vi "多反-初始化img句柄.vi"(11 "idx":i32) -> (3 "imgDFs":T2)   [LabVIEW 2018]
uses:
  <vilib>/vision/Image Controls.llb/IMAQ Image.ctl
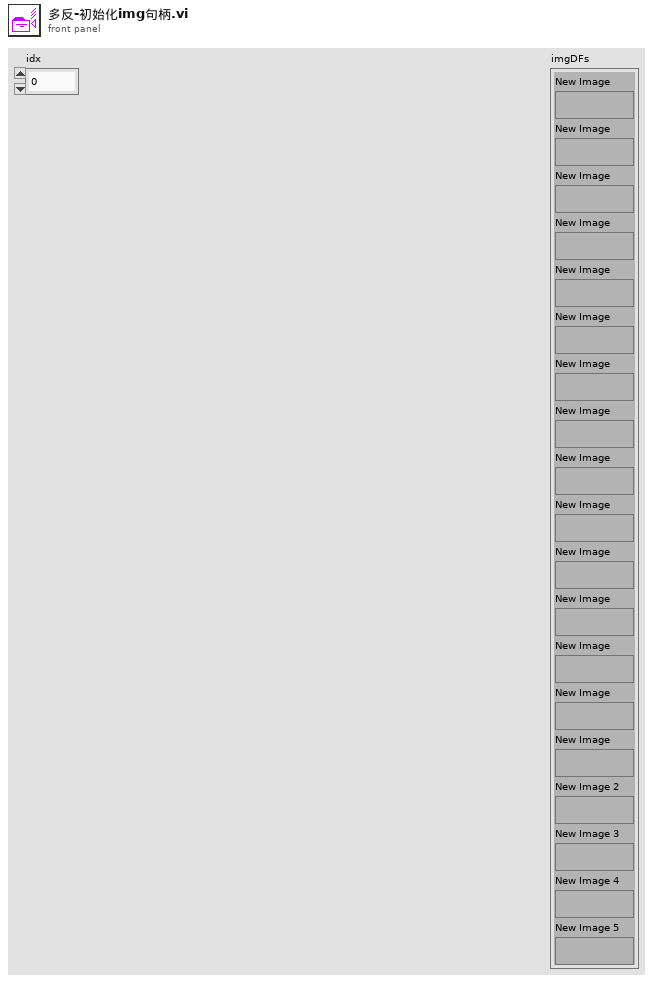
[diagram p1: front panel]
types:
  T1 = typedef "IMAQ Image.ctl" = refnum<image>
  T2 = cluster{"New Image":T1, "New Image":T1, "New Image":T1, "New Image":T1, "New Image":T1, "New Image":T1, "New Image":T1, "New Image":T1, "New Image":T1, "New Image":T1, "New Image":T1, "New Image":T1, "New Image":T1, "New Image":T1, "New Image":T1, "New Image 2":T1, "New Image 3":T1, "New Image 4":T1, "New Image 5":T1}
  T3 = typedef "Image Type" = u32
  T4 = cluster{"New Image":T1, "New Image":T1, "New Image":T1, "New Image":T1, "New Image":T1, "New Image":T1, "New Image":T1, "New Image":T1, "New Image":T1, "New Image":T1, "New Image":T1, "New Image":T1, "New Image":T1, "New Image":T1, "New Image":T1, "New Image":T1, "New Image":T1, "New Image":T1, "New Image":T1}
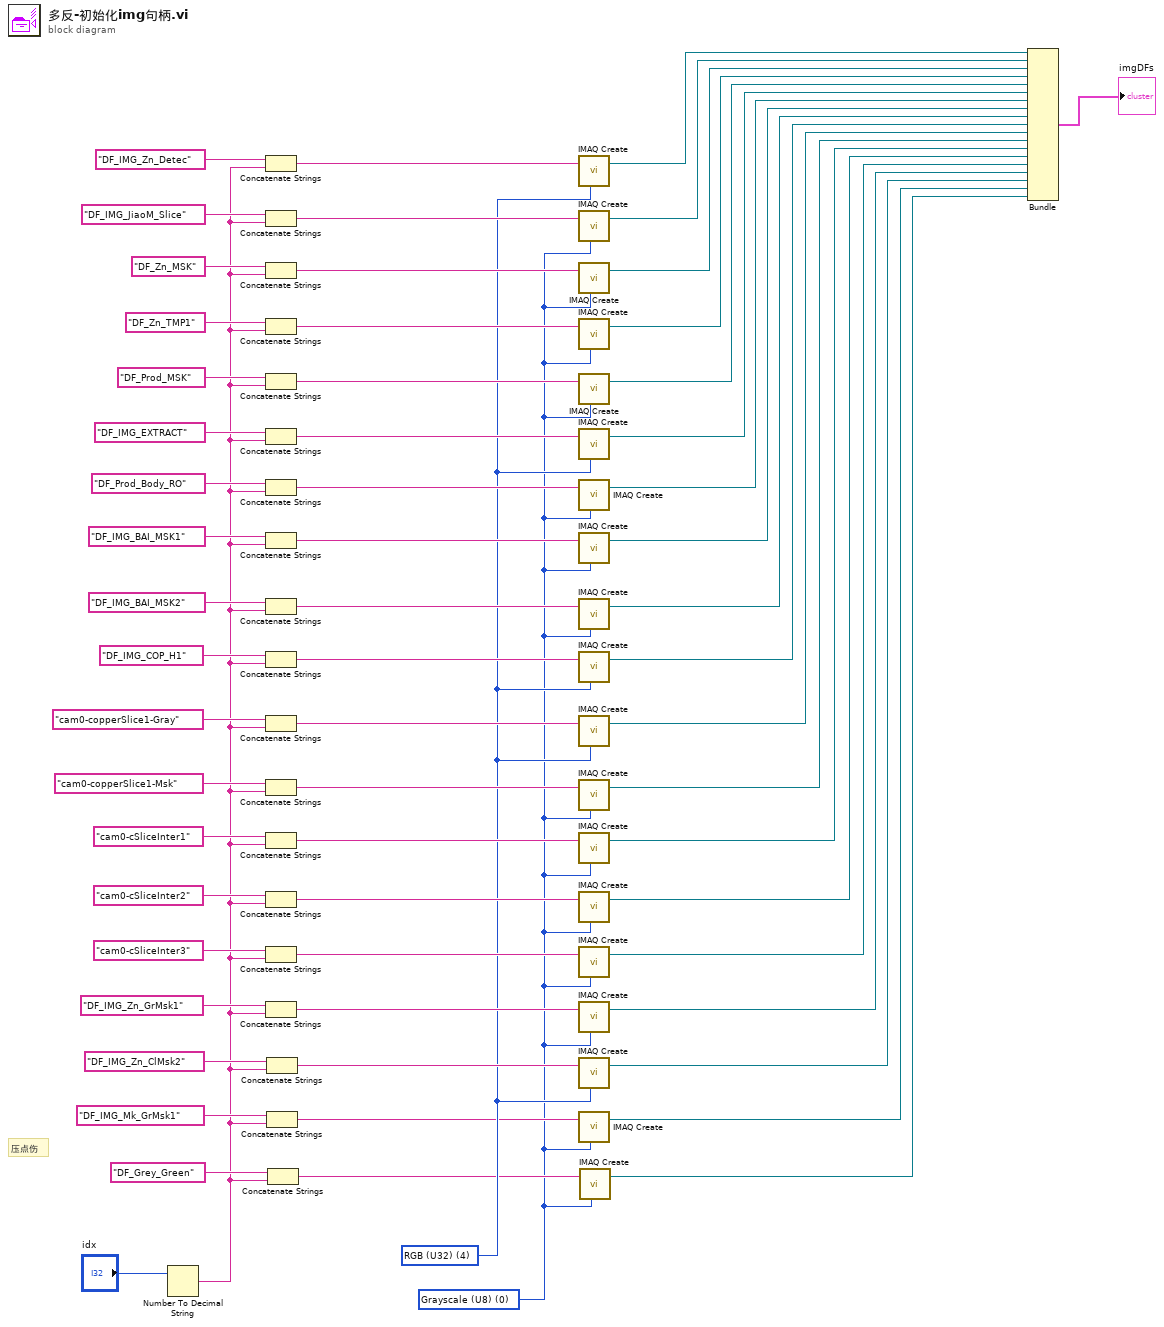
[diagram p0: block diagram]
diagram:
  w2 = T3 0 items=["Grayscale (U8)", "Grayscale (I16)", "Grayscale (SGL)", "Complex (CSG)", "RGB (U32)", "HSL (U32)", "RGB (U64)", "Grayscale (U16)"] ("Image Type")
  w11 = T3 4 items=["Grayscale (U8)", "Grayscale (I16)", "Grayscale (SGL)", "Complex (CSG)", "RGB (U32)", "HSL (U32)", "RGB (U64)", "Grayscale (U16)"] ("Image Type")
  # "压点伤"
  n1 = Number To Decimal String(number="idx") -> (decimal integer string=w3:string)  [unwired: 1 in]
  n2 = Concatenate Strings("DF_IMG_Zn_Detec" ("Image Name"), w3) -> (w61:string)
  n3 = Concatenate Strings("DF_IMG_JiaoM_Slice" ("Image Name"), w3) -> (w55:string)
  n4 = Concatenate Strings("DF_Zn_MSK" ("Image Name"), w3) -> (w53:string)
  n5 = Concatenate Strings("DF_Zn_TMP1" ("Image Name"), w3) -> (w51:string)
  n6 = Concatenate Strings("DF_Prod_MSK" ("Image Name"), w3) -> (w49:string)
  n7 = Concatenate Strings("DF_IMG_EXTRACT" ("Image Name"), w3) -> (w60:string)
  n8 = Concatenate Strings("DF_Prod_Body_RO" ("Image Name"), w3) -> (w57:string)
  n9 = Concatenate Strings("DF_IMG_BAI_MSK1" ("Image Name"), w3) -> (w48:string)
  n10 = Concatenate Strings("DF_IMG_BAI_MSK2" ("Image Name"), w3) -> (w47:string)
  n11 = Concatenate Strings("DF_IMG_COP_H1" ("Image Name"), w3) -> (w44:string)
  n12 = Concatenate Strings("cam0-copperSlice1-Gray" ("Image Name"), w3) -> (w42:string)
  n13 = Concatenate Strings("cam0-copperSlice1-Msk" ("Image Name"), w3) -> (w41:string)
  n14 = Concatenate Strings("cam0-cSliceInter1" ("Image Name"), w3) -> (w40:string)
  n15 = Concatenate Strings("cam0-cSliceInter2" ("Image Name"), w3) -> (w39:string)
  n16 = Concatenate Strings("cam0-cSliceInter3" ("Image Name"), w3) -> (w38:string)
  n17 = Concatenate Strings("DF_IMG_Zn_GrMsk1" ("Image Name"), w3) -> (w14:string)
  n18 = Concatenate Strings("DF_IMG_Zn_ClMsk2" ("Image Name"), w3) -> (w12:string)
  n19 = Concatenate Strings("DF_IMG_Mk_GrMsk1" ("Image Name"), w3) -> (w8:string)
  n20 = Concatenate Strings("DF_Grey_Green" ("Image Name"), w3) -> (w4:string)
  n21 = call "IMAQ Create"("Image Name"=w61, "Image Type"=w11) -> ("New Image"=w32:T1)  [unwired: 3 in, 1 out]
  n22 = call "IMAQ Create"("Image Name"=w55, "Image Type"=w2) -> ("New Image"=w31:T1)  [unwired: 3 in, 1 out]
  n23 = call "IMAQ Create"("Image Name"=w53, "Image Type"=w2) -> ("New Image"=w30:T1)  [unwired: 3 in, 1 out]
  n24 = call "IMAQ Create"("Image Name"=w51, "Image Type"=w2) -> ("New Image"=w29:T1)  [unwired: 3 in, 1 out]
  n25 = call "IMAQ Create"("Image Name"=w49, "Image Type"=w2) -> ("New Image"=w28:T1)  [unwired: 3 in, 1 out]
  n26 = call "IMAQ Create"("Image Name"=w60, "Image Type"=w11) -> ("New Image"=w27:T1)  [unwired: 3 in, 1 out]
  n27 = call "IMAQ Create"("Image Name"=w57, "Image Type"=w2) -> ("New Image"=w26:T1)  [unwired: 3 in, 1 out]
  n28 = call "IMAQ Create"("Image Name"=w48, "Image Type"=w2) -> ("New Image"=w25:T1)  [unwired: 3 in, 1 out]
  n29 = call "IMAQ Create"("Image Name"=w47, "Image Type"=w2) -> ("New Image"=w24:T1)  [unwired: 3 in, 1 out]
  n30 = call "IMAQ Create"("Image Name"=w44, "Image Type"=w11) -> ("New Image"=w23:T1)  [unwired: 3 in, 1 out]
  n31 = call "IMAQ Create"("Image Name"=w42, "Image Type"=w11) -> ("New Image"=w22:T1)  [unwired: 3 in, 1 out]
  n32 = call "IMAQ Create"("Image Name"=w41, "Image Type"=w2) -> ("New Image"=w21:T1)  [unwired: 3 in, 1 out]
  n33 = call "IMAQ Create"("Image Name"=w40, "Image Type"=w2) -> ("New Image"=w20:T1)  [unwired: 3 in, 1 out]
  n34 = call "IMAQ Create"("Image Name"=w39, "Image Type"=w2) -> ("New Image"=w19:T1)  [unwired: 3 in, 1 out]
  n35 = call "IMAQ Create"("Image Name"=w38, "Image Type"=w2) -> ("New Image"=w18:T1)  [unwired: 3 in, 1 out]
  n36 = call "IMAQ Create"("Image Name"=w14, "Image Type"=w2) -> ("New Image"=w10:T1)  [unwired: 3 in, 1 out]
  n37 = call "IMAQ Create"("Image Name"=w12, "Image Type"=w11) -> ("New Image"=w9:T1)  [unwired: 3 in, 1 out]
  n38 = call "IMAQ Create"("Image Name"=w8, "Image Type"=w2) -> ("New Image"=w6:T1)  [unwired: 3 in, 1 out]
  n39 = call "IMAQ Create"("Image Name"=w4, "Image Type"=w2) -> ("New Image"=w1:T1)  [unwired: 3 in, 1 out]
  n40 = Bundle("New Image"=w32, "New Image"=w31, "New Image"=w30, "New Image"=w29, "New Image"=w28, "New Image"=w27, "New Image"=w26, "New Image"=w25, "New Image"=w24, "New Image"=w23, "New Image"=w22, "New Image"=w21, "New Image"=w20, "New Image"=w19, "New Image"=w18, "New Image"=w10, "New Image"=w9, "New Image"=w6, "New Image"=w1) -> (→"imgDFs":T4)  [unwired: 1 in]
